vi "filterXYZero.vi"(10 "Filter Zero?":bool, 11 "Points":cluster{"x":dbl, "y":dbl}[](array[cluster])) -> (1 "Zero Removed":cluster{"x":dbl, "y":dbl}[](array[cluster]), 2 "Y":dbl[](array[numeric]), 3 "X":dbl[](array[numeric]))   [LabVIEW 2015]
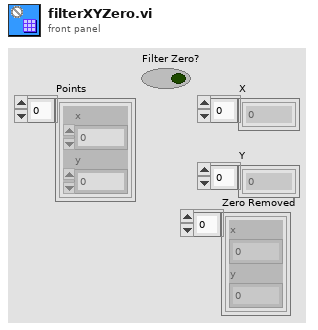
[diagram p1: front panel]
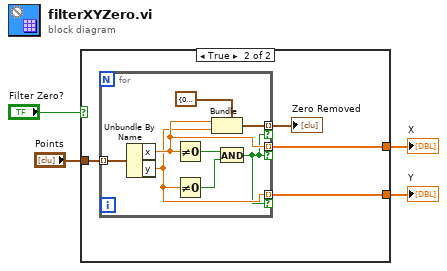
[diagram p0: block diagram]
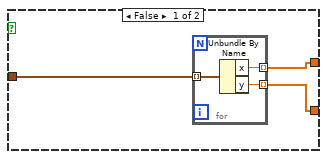
[diagram p2: hidden frame]
diagram:
  n1 = case shown="True" "Filter Zero?" {
    tunnel: [w5 w14] -> w4
    tunnel: [w6 w13] -> w3
    tunnel: "Points" -> [w7 w12]
    frame False {
      n2 = for {
        tunnel: w7 -> [w10] mode=indexing
        tunnel: [w9] -> w6 mode=indexing
        tunnel: [w8] -> w5 mode=indexing
        n3 = Unbundle By Name(w10) -> ("x"=w9:dbl, "y"=w8:dbl)
      }
    }
    frame True {
      n4 = for {
        tunnel: w12 -> [w22] mode=indexing
        tunnel: [w19] -> w13 mode=indexing if=w15
        tunnel: [w18] -> w14 mode=indexing if=w15
        tunnel: [w16] -> w11 mode=indexing if=w15
        n5 = Unbundle By Name(w22) -> ("x"=w19:dbl, "y"=w18:dbl)
        n6 = Not Equal To 0?(x=w19) -> (x != 0?=w20:bool)
        n7 = Not Equal To 0?(x=w18) -> (x != 0?=w21:bool)
        n8 = Bundle(cluster=cluster{"x":dbl, "y":dbl} {"x"=0.0, "y"=0.0} ("Cluster"), "x"=w19, "y"=w18) -> (w16:cluster{"x":dbl, "y":dbl})
        n9 = And(x=w20, y=w21) -> (x .and. y?=w15:bool)
      }
      "Zero Removed" <- w11
    }
  }
  "Y" <- w4
  "X" <- w3
